vi "Value.vi"(8 "Error In":errorcluster, 10 "Key":string, 11 "Non-Terminal In":refnum<class "NonTerminal.lvclass">) -> (0 "Error Out":errorcluster, 2 "Value":variant, 3 "Non-Terminal Out":refnum<class "NonTerminal.lvclass">)   [LabVIEW 2018, in "Toolkit.lvlib" / "Nodes.lvlib" / "NonTerminal.lvclass"]
uses:
  NonTerminal.lvclass
  NonTerminal.lvclass/NonTerminal.ctl
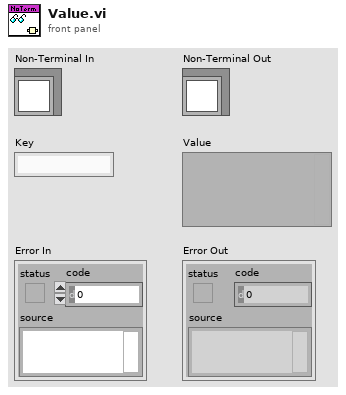
[diagram p1: front panel]
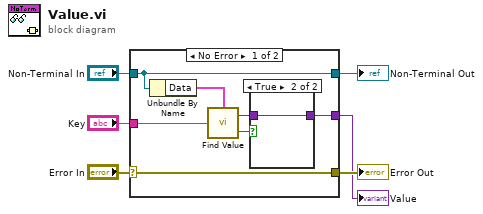
[diagram p0: block diagram]
diagram:
  n1 = case shown="No Error" "Error In" {
    selector: "Error In" -> [w11 w15]
    tunnel: "Non-Terminal In" -> [w8 w16]
    tunnel: [w8 w16] -> w4
    tunnel: [w11 w15] -> w3
    tunnel: "Key" -> [w12 _]
    tunnel: [w9 _] -> w1
    frame No Error {
      n2 = Unbundle By Name(w8) -> ("Data"=w13:cluster{"Key":string, "Value":variant}[])
      n3 = call "Find Value.vi"("Key"=w12, "Data"=w13) -> ("Value"=w10:variant, "Found?"=w7:bool)
      n4 = case shown="True" w7 {
        tunnel: w10 -> [_ w14]
        tunnel: [_ w14] -> w9
        frame False {
        }
        frame True {
        }
      }
    }
    frame Error {
    }
  }
  "Error Out" <- w3
  "Non-Terminal Out" <- w4
  "Value" <- w1
